vi "WirebirdLabs-JSON-Escape.vi"(1 "String":string) -> (0 "Escaped String":string)   [LabVIEW 2012]
panel:
  # "Inputs"
  # "Outputs"
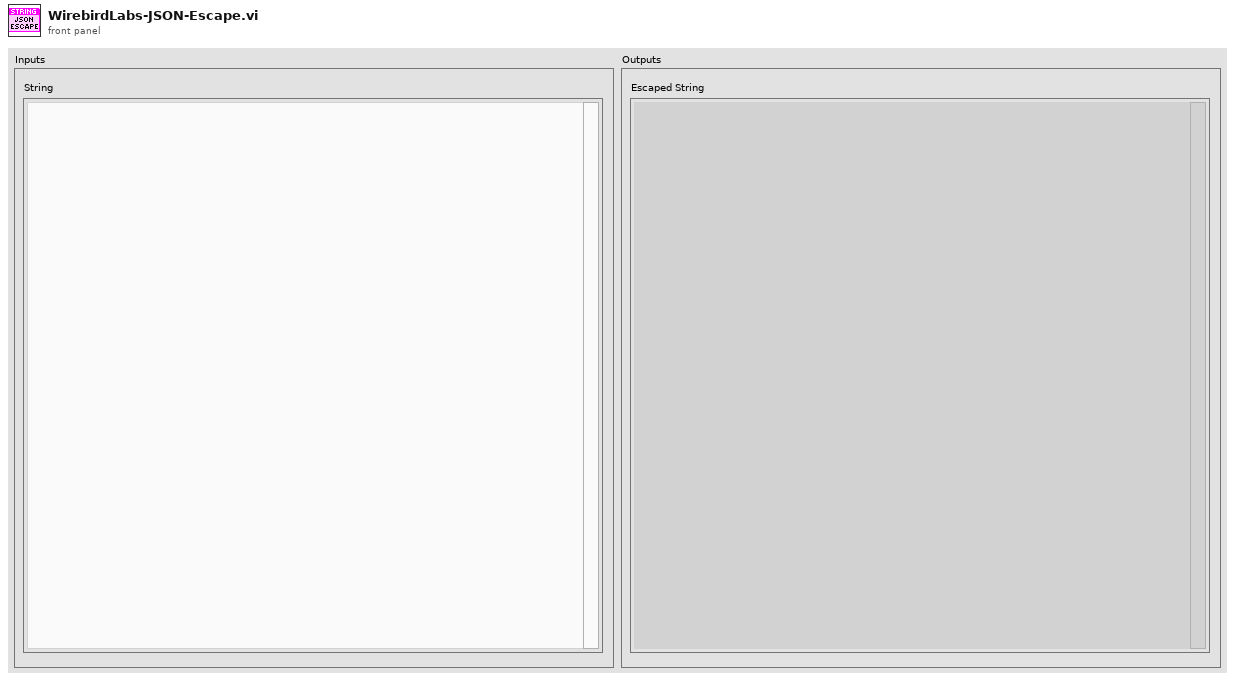
[diagram p1: front panel]
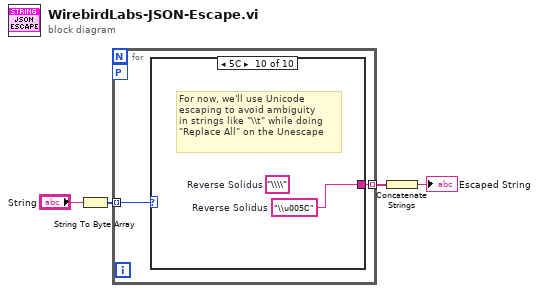
[diagram p0: block diagram]
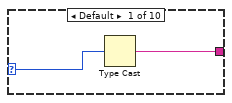
[diagram p2: hidden frame]
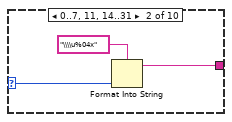
[diagram p3: hidden frame]
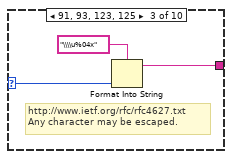
[diagram p4: hidden frame]
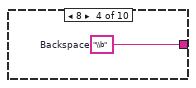
[diagram p5: hidden frame]
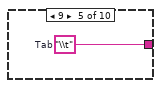
[diagram p6: hidden frame]
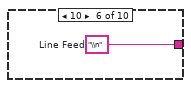
[diagram p7: hidden frame]
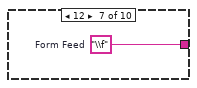
[diagram p8: hidden frame]
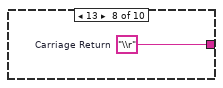
[diagram p9: hidden frame]
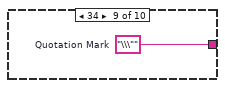
[diagram p10: hidden frame]
diagram:
  n1 = String To Byte Array(string="String") -> (unsigned byte array=w3:u8[])
  n2 = for {
    tunnel: w3 -> [w6] mode=indexing
    tunnel: [w5] -> w2 mode=indexing
    workers-P: _ -> [_]
    n3 = case shown="5C" w6 {
      selector: w6 -> [w8 w10 w13 _ _ _ _ _ _ _]
      tunnel: [w7 w9 w12 w15 w16 w17 w18 w19 w20 w21] -> w5
      frame Default {
        n4 = Type Cast(x=w8) -> (*(type *) &x=w7:string)  [unwired: 1 in]
      }
      frame 0..7, 11, 14..31 {
        n5 = Format Into String(format string="\\\\u%04x", w10) -> (resulting string=w9:string)  [unwired: 2 in, 1 out]
      }
      frame 91, 93, 123, 125 {
        # "http://www.ietf.org/rfc/rfc4627.txt\nAny character may be escaped."
        n6 = Format Into String(format string="\\\\u%04x", w13) -> (resulting string=w12:string)  [unwired: 2 in, 1 out]
      }
      frame 8 {
        w15 = "\\b"  # Backspace
      }
      frame 9 {
        w16 = "\\t"  # Tab
      }
      frame 10 {
        w17 = "\\n"  # Line Feed
      }
      frame 12 {
        w18 = "\\f"  # Form Feed
      }
      frame 13 {
        w19 = "\\r"  # Carriage Return
      }
      frame 34 {
        w20 = "\\\""  # Quotation Mark
      }
      frame 92 {
        w21 = "\\u005C"  # Reverse Solidus
        (unwired) "\\\\"  # Reverse Solidus
        # "For now, we'll use Unicode\nescaping to avoid ambiguity\nin strings like \"\\\\t\" while doing\n\"Replace All\" on the Unescape"
      }
    }
  }
  n7 = Concatenate Strings(w2) -> (→"Escaped String":string)
